vi "Update Comm Link.vi"(8 "error in (no error)":errorcluster, 10 "Comms/Python Link":bool, 11 "Telemetry Data in":T1) -> (0 "error out":errorcluster, 3 "Telemetry Data out":T1)   [LabVIEW 2026, in "TCP.lvlib"]
uses:
  TCP.lvlib
  Controls/Telemetry_Data_Type.ctl
  Controls/Channels.ctl
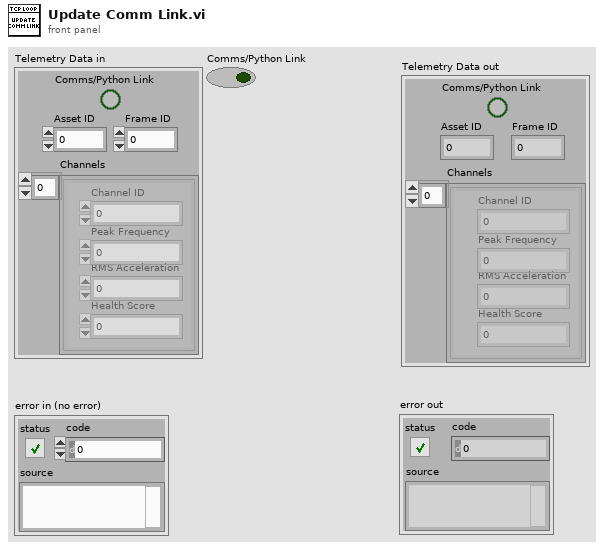
[diagram p1: front panel]
types:
  T1 = typedef "Telemetry_Data_Type.ctl" = cluster{"asset_id":i32, "frame_id":i32, "channels":T2, "comms/python link":bool}
  T2 = typedef "Channels.ctl" = cluster{"channel_id":dbl, "peak_frequency":dbl, "rms_acceleration":dbl, "health_score":dbl}[]
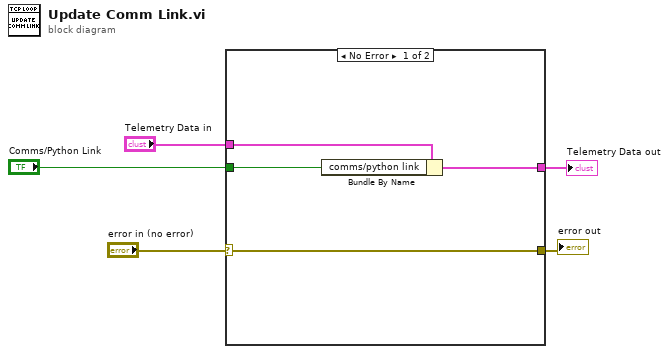
[diagram p0: block diagram]
diagram:
  n1 = case shown="No Error" "error in (no error)" {
    selector: "error in (no error)" -> [w9 w10]
    tunnel: [w9 w10] -> w4
    tunnel: "Telemetry Data in" -> [w8 w11]
    tunnel: [w7 w11] -> w2
    tunnel: "Comms/Python Link" -> [w6 _]
    frame No Error {
      n2 = Bundle By Name(cluster=w8, "comms/python link"=w6) -> (w7:T1)
    }
    frame Error {
    }
  }
  "error out" <- w4
  "Telemetry Data out" <- w2
